vi "ReadSerial_Basic_JE_001.vi"() -> ()   [LabVIEW 2011]
uses:
  <vilib>/Instr/_visa.llb/VISA Configure Serial Port (Serial Instr).vi
panel:
  out "size(s)":i32
  out "Waveform Chart":T1(graph)
  in  "N data blocks to read":dbl=1.0
  in  "byte order (0:big-endian, network order) 2":T2(ring)
  in  "file (use dialog)":path
  out "ascii code u8":i32
  out "concatenated string":string
  out "Graphical Representation of Data":u16[](graph)
  in  "byte order (0:big-endian, network order)":T2(ring)
  out "strlen":i32
  in  "VISA resource name":refnum<visa-resource-name>
  out "Nbytes written from Teensy to Serial Port":u32
  in  "baud rate (9600)":u32=9600
  in  "data bits (8)":u16=8 min=5 max=8 step=1
  in  "stop bits (10: 1 bit)":u16(ring)=10 items=["1.0"=10, "1.5"=15, "2.0"=20]
  in  "flow control (0:none)":u16(ring) items=["None", "XON/XOFF", "RTS/CTS", "XON/XOFF & RTS/CTS", "DTR/DSR", "XON/XOFF & DTR/DSR"]
  in  "parity (0:none)":enum16{"None", "Odd", "Even", "Mark", "Space"}(ring)
  in  "stop":bool
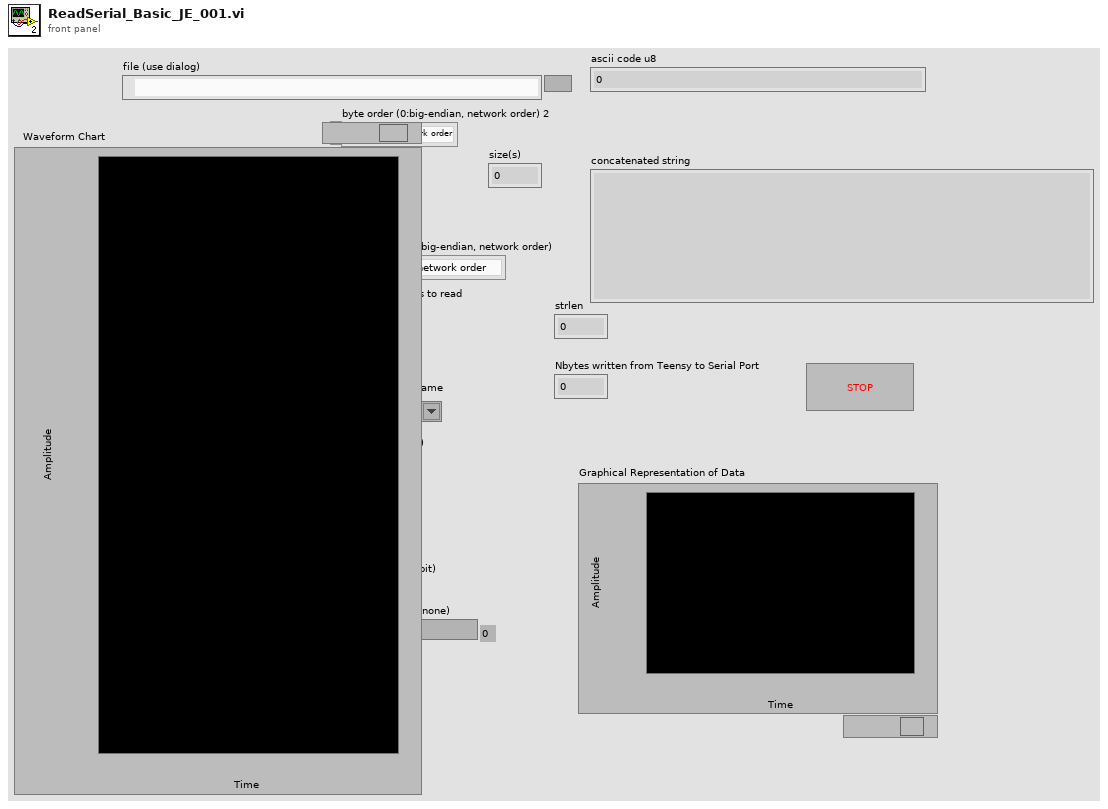
[diagram p1: front panel]
types:
  T1 = cluster{"[0]":u16, "[1]":u16, "[2]":u16, "[3]":u16, "[4]":u16, "[5]":u16, "[6]":u16, "[7]":u16, "[8]":u16, "[9]":u16, "[10]":u16, "[11]":u16, "[12]":u16, "[13]":u16, "[14]":u16, "[15]":u16, "[16]":u16, "[17]":u16, "[18]":u16, "[19]":u16, "[20]":u16, "[21]":u16, "[22]":u16, "[23]":u16, "[24]":u16, "[25]":u16, "[26]":u16, "[27]":u16, "[28]":u16, "[29]":u16, "[30]":u16, "[31]":u16}
  T2 = enum16{"big-endian, network order", "native, host order", "little-endian"}
  T3 = enum16{"open", "replace", "create", "open or create", "replace or create", "replace or create with confirmation"}
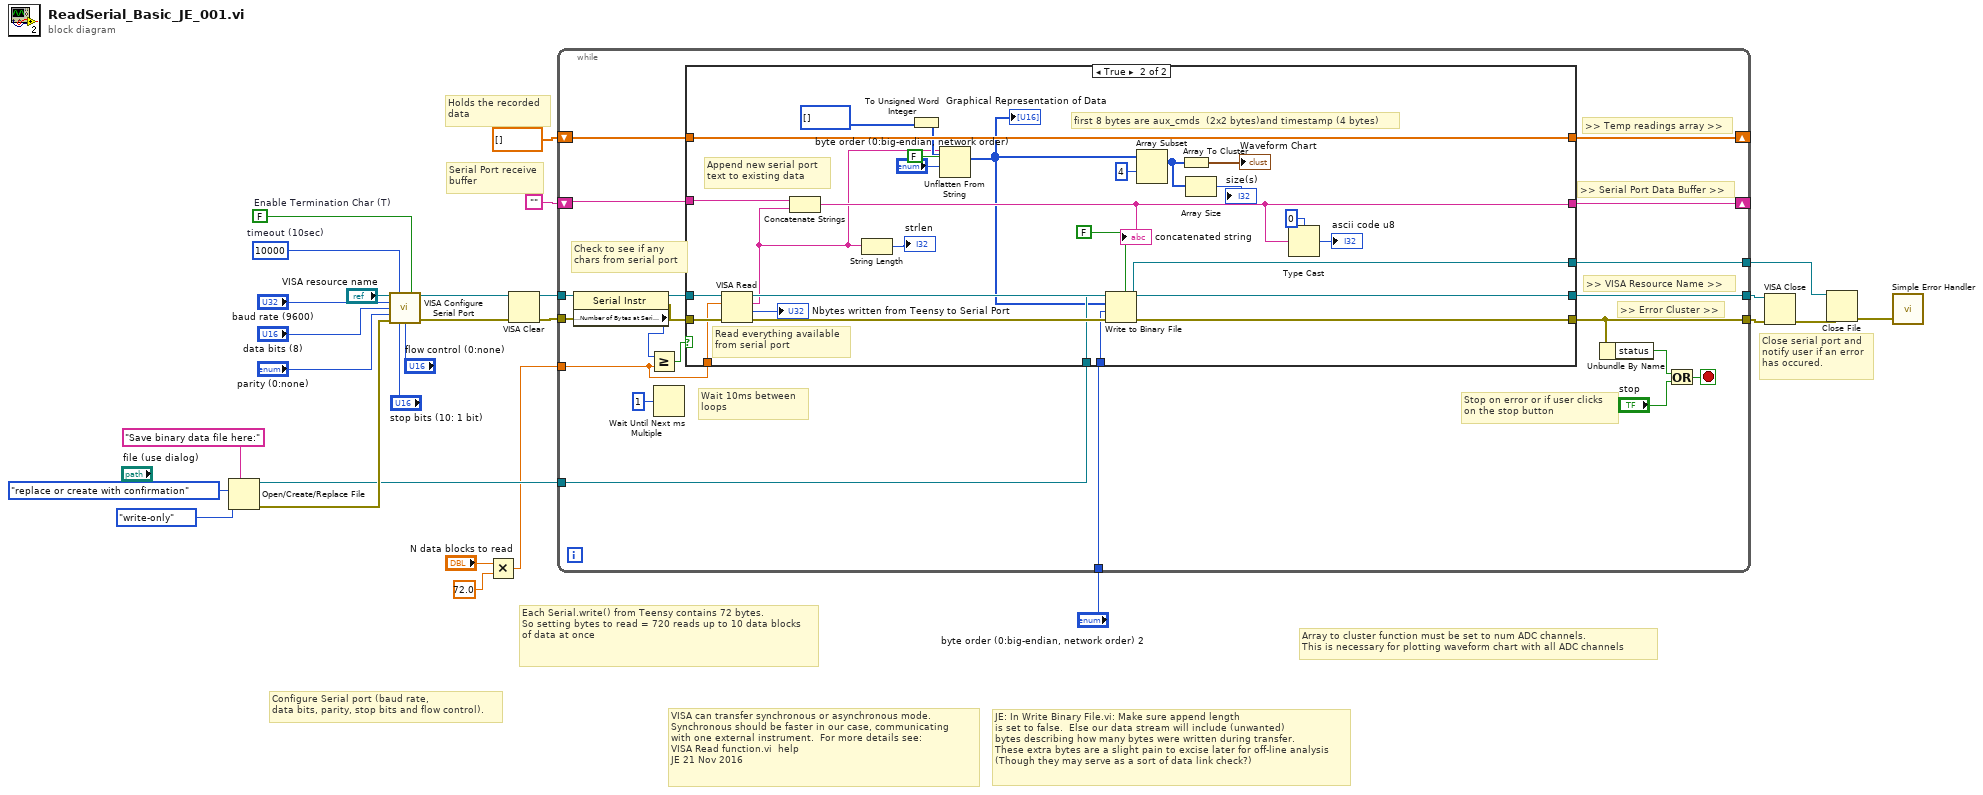
[diagram p0: block diagram]
diagram:
  w25 = FALSE  # Enable Termination Char (T)
  w26 = u32 10000  # timeout (10sec)
  # "Array to cluster function must be set to num ADC channels. \nThis is necessary for plotting waveform chart with all ADC channels"
  # "Each Serial.write() from Teensy contains 72 bytes.\nSo setting bytes to read = 720 reads up to 10 data blocks\nof data at once"
  # "JE: In Write Binary File.vi: Make sure append length \nis set to false.  Else our data stream will include (unwanted)\nbytes describing how many bytes were written during transfer.\nThese extra bytes are a slight pain to excise later for off-line analysis\n(Though they may serve as a sort of data link check?)"
  # "VISA can transfer synchronous or asynchronous mode.\nSynchronous should be faster in our case, communicating\nwith one external instrument.  For more details see: \nVISA Read function.vi  help \nJE 21 Nov 2016"
  # "Close serial port and\nnotify user if an error\nhas occured."
  # "Serial Port receive\nbuffer"
  # "Holds the recorded\ndata"
  # "Configure Serial port (baud rate,\ndata bits, parity, stop bits and flow control)."
  n1 = Open/Create/Replace File(prompt="Save binary data file here:" ("prompt (Choose or enter file path)"), operation (0:open)=T3."replace or create with confirmation", access (0:read/write)=enum16{"read/write", "read-only", "write-only"}."write-only") -> (refnum out=w8:refnum<file>, error out=w9:errorcluster)  [unwired: 3 in, 1 out]
  n2 = call-poly "VISA Configure Serial Port"("VISA resource name"="VISA resource name", "timeout (10sec)"=w26, "Enable Termination\nChar (T)"=w25, "baud rate (9600)"="baud rate (9600)", "data bits (8)"="data bits (8)", "parity (0:none)"="parity (0:none)", "error in (no error)"=w9, "stop bits (10: 1 bit)"="stop bits (10: 1 bit)", "flow control (0:none)"="flow control (0:none)") -> ("VISA resource name out"=w23:refnum<visa-resource-name>, "error out"=w24:errorcluster)  [unwired: 5 in]
  n3 = Multiply(x="N data blocks to read", y=72.0) -> (x*y=w1:dbl)
  n4 = VISA Clear(VISA resource name=w23, error in (no error)=w24) -> (VISA resource name out=w21:refnum<visa-resource-name>, error out=w20:errorcluster)
  n5 = while {
    tunnel: [w41] -> w28
    tunnel: [w48] -> w27
    shift-right: [w35] -> _
    shift-left: "" -> [w43]
    tunnel: w21 -> [w45]
    tunnel: w20 -> [w44]
    shift-right: [w37] -> _
    shift-left: dbl[] [] -> [w36]
    tunnel: w8 -> [w32]
    tunnel: [w31] -> w5
    tunnel: "byte order (0:big-endian, network order) 2" -> [w30]
    tunnel: w1 -> [w29]
    stop <- w40 stop-if-true
    # "Wait 10ms between \nloops"
    # "Stop on error or if user clicks \non the stop button"
    # ">> Error Cluster >>"
    # ">> VISA Resource Name >>"
    # ">> Temp readings array >>"
    # ">> Serial Port Data Buffer >>"
    # "Check to see if any\nchars from serial port"
    n6 = property class="Serial Instr"(reference=w45, error in=w44) -> (reference out=w47:refnum<visa-resource-name>, error out=w46:errorcluster, "Serial Settings:Number of Bytes at Serial Port"=w34:u32)
    n7 = Greater Or Equal?(x=w34, y=w29) -> (x >= y?=w33:bool)
    n8 = Wait Until Next ms Multiple(millisecond multiple=u32 1) -> ()  [unwired: 1 out]
    n9 = case shown="True" w33 {
      tunnel: [w52 w65] -> w41
      tunnel: [w53 w80] -> w48
      tunnel: w47 -> [w53 w79]
      tunnel: w46 -> [w52 w78]
      tunnel: w43 -> [w51 w77]
      tunnel: [w51 w71] -> w35
      tunnel: [w50 w74] -> w37
      tunnel: w36 -> [w50 w74]
      tunnel: w29 -> [_ w76]
      tunnel: w32 -> [w49 w64]
      tunnel: [w49 w63] -> w31
      tunnel: w30 -> [_ w59]
      frame False {
        # "No data in from serial port - Nothing to do."
      }
      frame True {
        # "first 8 bytes are aux_cmds  (2x2 bytes)and timestamp (4 bytes)"
        # "Append new serial port\ntext to existing data"
        # "Read everything available\nfrom serial port"
        n10 = VISA Read(VISA resource name=w79, byte count=w76, error in (no error)=w78) -> (VISA resource name out=w80:refnum<visa-resource-name>, read buffer=w67:string, return count=→"Nbytes written from Teensy to Serial Port":u32, error out=w66:errorcluster)
        n11 = Concatenate Strings(w77, w67) -> (w71:string)
        "concatenated string" <- w71
        n12 = String Length(string=w67) -> (length=→"strlen":i32)
        n13 = To Unsigned Word Integer(number=i16[] []) -> (unsigned 16bit integer=w68:u16[])
        n14 = Unflatten From String(type=w68, binary string=w67, data includes array or string size? (T)=FALSE, byte order (0:big-endian, network order)="byte order (0:big-endian, network order)") -> (value=w58:u16[])  [unwired: 1 in, 2 out]
        "Graphical Representation of Data" <- w58
        n15 = Write to Binary File(file (use dialog)=w64, data=w58, error in=w66, 5:FALSE ("prepend array or string size? (T)"), 9:w59) -> (refnum out=w63:refnum<file>, error out=w65:errorcluster)  [unwired: 1 in, 1 out]
        n16 = Array Subset(array=w58, index=4) -> (w55:u16[])  [unwired: 1 in]
        n17 = Array To Cluster(array=w55) -> (cluster=→"Waveform Chart":T1)
        n18 = Array Size(array=w55) -> (size(s)=→"size(s)":i32)
        n19 = Type Cast(type=0, x=w71) -> (*(type *) &x=→"ascii code u8":i32)
      }
    }
    n20 = Unbundle By Name(w41) -> ("status"=w39:bool)
    n21 = Or(x=w39, y="stop") -> (x .or. y?=w40:bool)
  }
  n22 = VISA Close(VISA resource name=w27, error in (no error)=w28) -> (error out=w7:errorcluster)
  n23 = Close File(refnum=w5, error in=w7) -> (error out=w6:errorcluster)  [unwired: 1 out]
  n24 = call <vilib>:"Simple Error Handler.vi"("error in (no error)"=w6) -> ()  [unwired: 4 in, 5 out]
